vi "Write Logger.vi"(8 "error in (no error)":errorcluster, 10 "Logger.lvclass":refnum<class "Logger.lvclass">, 11 "Template Module in":refnum<class "Template Module.lvclass">) -> (0 "error out":errorcluster, 3 "Template Module out":refnum<class "Template Module.lvclass">)   [LabVIEW 2019, in "Template Module.lvclass"]
uses:
  Template Module.lvclass
  Loggers/Logger/Logger.lvclass
  Template Module.lvclass/Template Module.ctl
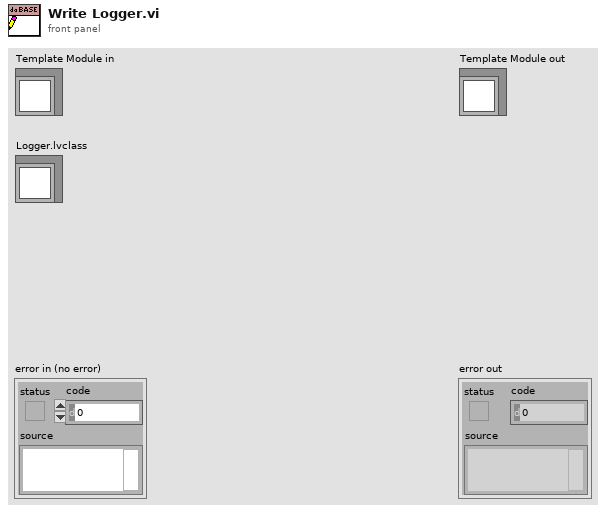
[diagram p1: front panel]
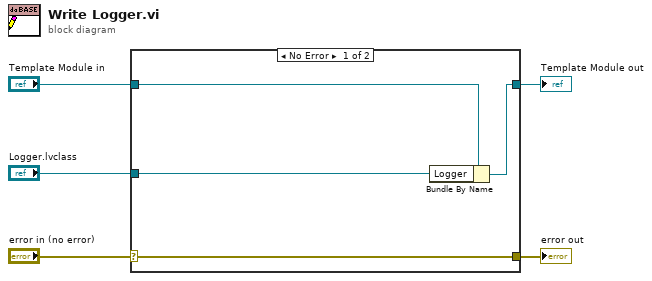
[diagram p0: block diagram]
diagram:
  n1 = case shown="No Error" "error in (no error)" {
    selector: "error in (no error)" -> [w9 w10]
    tunnel: [w9 w10] -> w4
    tunnel: [w7 w11] -> w2
    tunnel: "Template Module in" -> [w8 w11]
    tunnel: "Logger.lvclass" -> [w6 _]
    frame No Error {
      n2 = Bundle By Name(cluster=w8, "Logger"=w6) -> (w7:refnum<class "Template Module.lvclass">)
    }
    frame Error {
    }
  }
  "error out" <- w4
  "Template Module out" <- w2
